vi "Get Bool By Name.vi"(0 "name":string, 2 "Digital Values":T1) -> (7 "result":bool, 9 "found?":bool)   [LabVIEW 2013]
uses:
  controls/Digital Values.ctl
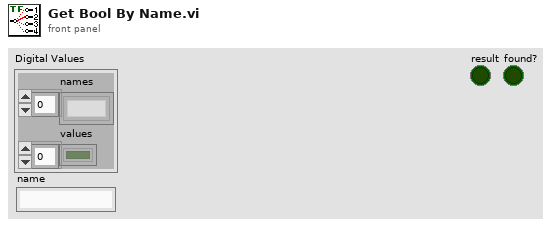
[diagram p1: front panel]
types:
  T1 = typedef "Digital Values.ctl" = cluster{"names":string[], "values":bool[]}
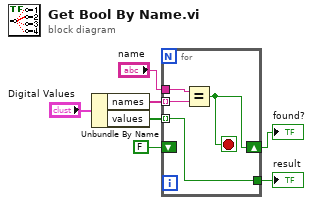
[diagram p0: block diagram]
diagram:
  n1 = Unbundle By Name("Digital Values") -> ("names"=w6:string[], "values"=w5:bool[])
  n2 = for {
    tunnel: w6 -> [w9] mode=indexing
    tunnel: w5 -> [w11] mode=indexing
    tunnel: [w11] -> w3
    tunnel: "name" -> [w10]
    shift-right: [w8] -> w1
    shift-left: FALSE -> [_]
    stop <- w8 stop-if-true
    n3 = Equal?(x=w10, y=w9) -> (x = y?=w8:bool)
  }
  "result" <- w3
  "found?" <- w1
